vi "Write Data - All tubes.vi"(9 "Array":dbl[](array[numeric]), 10 "Barcodes":string[](array[string]), 11 "Channel Number":string) -> ()   [LabVIEW 2020]
uses:
  <vilib>/Utility/file.llb/Write Delimited Spreadsheet (string).vi
  <vilib>/Utility/file.llb/Write Delimited Spreadsheet (DBL).vi
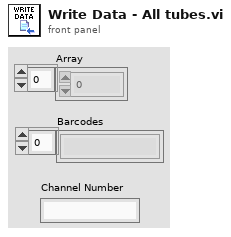
[diagram p1: front panel]
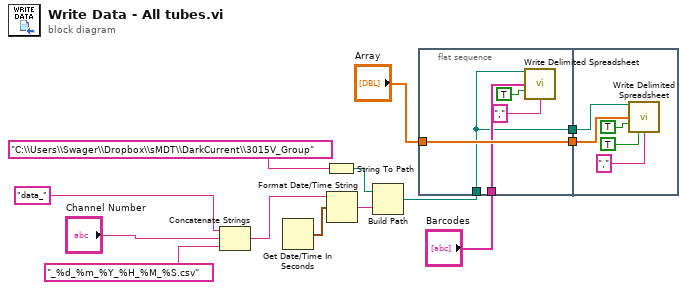
[diagram p0: block diagram]
diagram:
  n1 = Concatenate Strings("data_", "Channel Number", "_%d_%m_%Y_%H_%M_%S.csv" ("string")) -> (w2:string)
  n2 = Get Date/Time In Seconds() -> (seconds since 1Jan1904=w10:timestamp)
  n3 = String To Path(string="C:\\Users\\Swager\\Dropbox\\sMDT\\DarkCurrent\\3015V_Group") -> (path=w9:path)
  n4 = Format Date/Time String(time format string (%c)=w2, seconds (now)=w10) -> (date/time string=w11:string)  [unwired: 1 in]
  n5 = Build Path(base path=w9, name or relative path=w11) -> (appended path=w7:path)
  n6 = flat-sequence {
    tunnel: [w18] -> w13
    tunnel: w7 -> [w14]
    tunnel: "Barcodes" -> [w17]
    tunnel: "Array" -> [w18]
    tunnel: [w14] -> w6
    tunnel: w13 -> [w20]
    tunnel: w6 -> [w21]
    frame #0 {
      n7 = call-poly <vilib>:"Write Delimited Spreadsheet.vi"("file path (dialog if empty)"=w14, "1D data"=w17, "append to file? (new file:F)"=TRUE, "delimiter (\\t)"=",") -> ()  [unwired: 10 in, 2 out]
    }
    frame #1 {
      n8 = call-poly <vilib>:"Write Delimited Spreadsheet.vi"("file path (dialog if empty)"=w21, "1D data"=w20, "append to file? (new file:F)"=TRUE, "transpose? (no:F)"=TRUE, "delimiter (\\t)"=",") -> ()  [unwired: 9 in, 2 out]
    }
  }
